vi "ITC503_set_values.vi"(4 "ITC503-Status-Monitor":T1={"Temperatur (K)"=0.0, "Heater (%)"=0.0, "NV (%)"=0.0, "Heater Manual"=FALSE, "NV Manual"=FALSE, "Valid?"=FALSE, "Heater (%) Display"=3.4572, "NV (%) Display"=3.4572, "Sample 3"=0.0, "Sample 2"=0.0, "Sweep-State"=FALSE, "Auto PID"=FALSE, "Setpoint-Sweep"=0.0, "Sample 1"=0.0, "Channel 1"=FALSE, "Channel 2"=FALSE, "Channel 3"=FALSE} {"NV (%) Display" format="%4_5f"; "Heater (%) Display" format="%4_5f"; "NV (%)" scale=0.0..100.0; "Heater (%)" scale=0.0..100.0}, 5 "System Monitor Variables (in)":T2) -> (1 "System Monitor Variables (out)":T2)   [LabVIEW 2019]
uses:
  Global/Global Variables/System Monitor Cluster.ctl
  ITC503/ITC503_Status.ctl
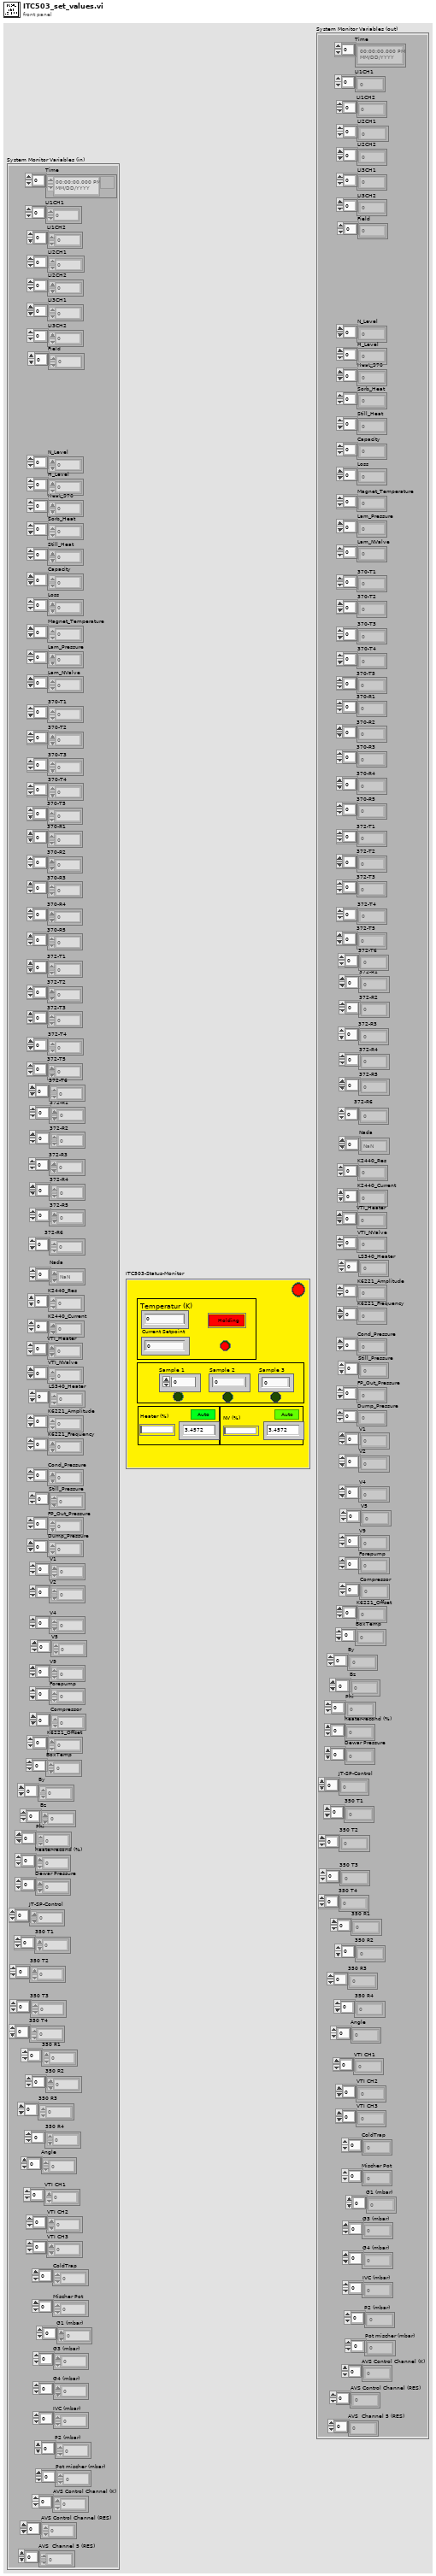
[diagram p1: front panel]
types:
  T1 = typedef "ITC503_Status.ctl" = cluster{"Temperatur (K)":dbl, "Heater (%)":dbl, "NV (%)":dbl, "Heater Manual":bool, "NV Manual":bool, "Valid?":bool, "Heater (%) Display":dbl, "NV (%) Display":dbl, "Sample 3":dbl, "Sample 2":dbl, "Sweep-State":bool, "Auto PID":bool, "Setpoint-Sweep":dbl, "Sample 1":dbl, "Channel 1":bool, "Channel 2":bool, "Channel 3":bool}
  T2 = typedef "System Monitor Cluster.ctl" = cluster{"Time":timestamp[], "LI1CH1":dbl[], "LI1CH2":dbl[], "LI2CH1":dbl[], "LI2CH2":dbl[], "LI3CH1":dbl[], "LI3CH2":dbl[], "Field":dbl[], "N_Level":dbl[], "H_Level":dbl[], "Heat_370":dbl[], "Sorb_Heat":dbl[], "Still_Heat":dbl[], "Capacity":dbl[], "Loss":dbl[], "Magnet_Temperature":dbl[], "Lam_Pressure":dbl[], "Lam_NValve":dbl[], "370-T1":dbl[], "370-T2":dbl[], "370-T3":dbl[], "370-T4":dbl[], "370-T5":dbl[], "370-R1":dbl[], "370-R2":dbl[], "370-R3":dbl[], "370-R4":dbl[], "370-R5":dbl[], "372-T1":dbl[], "372-T2":dbl[], "372-T3":dbl[], "372-T4":dbl[], "372-T5":dbl[], "372-T6":dbl[], "372-R1":dbl[], "372-R2":dbl[], "372-R3":dbl[], "372-R4":dbl[], "372-R5":dbl[], "372-R6":dbl[], "Nada":dbl[], "K2440_Res":dbl[], "K2440_Current":dbl[], "VTI_Heater":dbl[], "VTI_NValve":dbl[], "LS340_Heater":dbl[], "K6221_Amplitude":dbl[], "K6221_Frequency":dbl[], "Cond_Pressure":dbl[], "Still_Pressure":dbl[], "FP_Out_Pressure":dbl[], "Dump_Pressure":dbl[], "V1":dbl[], "V2":dbl[], "V4":dbl[], "V5":dbl[], "V9":dbl[], "Forepump":dbl[], "Compressor":dbl[], "K6221_Offset":dbl[], "BoxTemp":dbl[], "By":dbl[], "Bz":dbl[], "Phi":dbl[], "heater-recond (%)":dbl[], "Dewar Pressure ":dbl[], "JT-SP-Control":dbl[], "350 T1":dbl[], "350 T2":dbl[], "350 T3":dbl[], "350 T4":dbl[], "350 R1":dbl[], "350 R2":dbl[], "350 R3":dbl[], "350 R4":dbl[], "Angle":dbl[], "VTI CH1":dbl[], "VTI CH2":dbl[], "VTI CH3":dbl[], "ColdTrap":dbl[], "Mischer Pot":dbl[], "G1 (mbar)":dbl[], "G3 (mbar) ":dbl[], "G4 (mbar)":dbl[], "IVC (mbar)":dbl[], "P2 (mbar) ":dbl[], "Pot mischer (mbar)":dbl[], "AVS Control Channel (K)":dbl[], "AVS Control Channel (RES)":dbl[], "AVS  Channel 5 (RES) ":dbl[]}
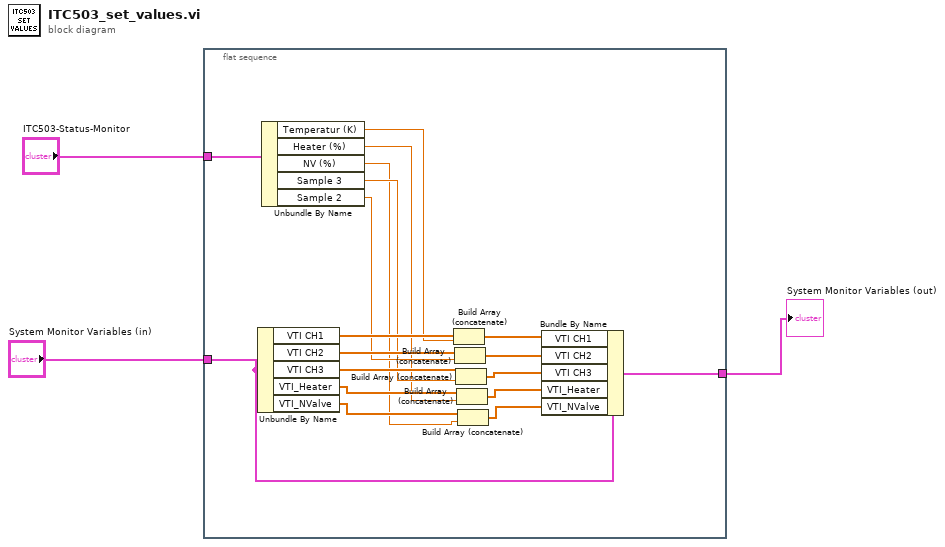
[diagram p0: block diagram]
diagram:
  n1 = flat-sequence {
    tunnel: "ITC503-Status-Monitor" -> [w21]
    tunnel: "System Monitor Variables (in)" -> [w20]
    tunnel: [w4] -> w1
    frame #0 {
      n2 = Unbundle By Name(w20) -> ("VTI CH1"=w19:dbl[], "VTI CH2"=w16:dbl[], "VTI CH3"=w14:dbl[], "VTI_Heater"=w12:dbl[], "VTI_NValve"=w10:dbl[])
      n3 = Unbundle By Name(w21) -> ("Temperatur (K)"=w18:dbl, "Heater (%)"=w11:dbl, "NV (%)"=w9:dbl, "Sample 3"=w13:dbl, "Sample 2"=w15:dbl)
      n4 = Build Array (concatenate)(w19, w18) -> (w17:dbl[])
      n5 = Build Array (concatenate)(w16, w15) -> (w8:dbl[])
      n6 = Build Array (concatenate)(w14, w13) -> (w7:dbl[])
      n7 = Build Array (concatenate)(w12, w11) -> (w6:dbl[])
      n8 = Build Array (concatenate)(w10, w9) -> (w5:dbl[])
      n9 = Bundle By Name(cluster=w20, "VTI CH1"=w17, "VTI CH2"=w8, "VTI CH3"=w7, "VTI_Heater"=w6, "VTI_NValve"=w5) -> (w4:T2)
    }
  }
  "System Monitor Variables (out)" <- w1
